vi "Udp Tester ffwd.vi"() -> ()   [LabVIEW 2014]
uses:
  <vilib>/addons/control/pid/pid.llb/PID Lead-Lag (DBL).vi
  <vilib>/addons/control/pid/pid.llb/PID (DBL).vi
  <vilib>/addons/control/pid/pid.llb/PID Percentage to EGU (DBL).vi
  <vilib>/FPGAPlugInAG/myRIO-1900/niLvFpga_Open_myRIO-1900.vi
  <vilib>/rvi/interface/common/dynamic/niFpgaDynamicAddResources.vi
  <vilib>/Utility/error.llb/Error Cluster From Error Code.vi
  <vilib>/rvi/errors/niLvFpgaAdjustHostInterfaceError.vi
  <vilib>/FPGAPlugInAG/Dynamic/niLvFpga_Close_Dynamic.vi
  <vilib>/rvi/interface/nirviOpenFPGA/nirviOpenFPGA.xnode
  FPGA Bitfiles/Test_FPGATarget_CurrentControl_60eBuCSPTsI.lvbitx
  Current Control.vi
  <vilib>/rvi/interface/nirviReadWriteControl/nirviReadWriteControl.xnode
  <vilib>/rvi/interface/nirviCloseFPGA/nirviCloseFPGA.xnode
  <vilib>/rvi/interface/Simulation/niFpgaSimulationCallBeginRW.vi
  <vilib>/Utility/file.llb/Write To Spreadsheet File (I64).vi
  <vilib>/addons/control/pid/NI_PID_pid.lvlib
  <vilib>/ptbypt/NI_PtbyPt.lvlib
  NiFpgaLv.dll
panel:
  in  "output range":cluster{"output high":dbl, "output low":dbl}={"output high"=100.0, "output low"=-100.0} {"output low" format="%.2f"; "output high" format="%.2f"}
  out "SP1:":dbl(slide)=40.87020302841148 min=0.0 max=0.0 scale=0.0..100.0
  in  "Feedforward\nLag Time (min)":dbl(slide)=0.9102981779915218 scale=0.01..10.0
  out "SP and PV":cluster{"Plant Output":dbl, "SP:":dbl}(graph)
  out "MV (mA)":dbl(graph)=20.39115328927357
  in  "Loop Cycle":i32
  in  "Tab Control":enum32{"Profile", "Diagram"}(tab)
  out "Inflow Profile Graph":cluster{dbl, dbl}[](graph)
  in  "Apply Inflow Profile":bool=TRUE
  in  "Constant Flow (%)":dbl=40.0
  in  "Inflow Profile":cluster{"time (s)":dbl, "setpoint":dbl}[](array[cluster])=[{"time (s)"=0.0, "setpoint"=40.0}, {"time (s)"=10.0, "setpoint"=40.0}, {"time (s)"=10.0, "setpoint"=60.0}, {"time (s)"=20.0, "setpoint"=60.0}]
  out "FT Valve":dbl(knob)=84.28886007445381 scale=0.0..190.0
  out "control valve":dbl=86.66603993277398 format="%.2f"
  out "Valve":bool
  out "Pump":bool=TRUE
  out "Bladder Tank":dbl(slide)=49.279730305904245 scale=0.0..100.0 scale format="%.2f"
  out "FT":dbl(knob)=84.28886007445381 scale=0.0..100.0
  out "PV 1":dbl=49.279730305904245
  in  "Stop":bool
  in  "PID parameters (LC)":T1={"Kc"=-20.0, "Ti (min)"=0.1, "Td (min)"=0.0} {"Td (min)" format="%#.6f"; "Ti (min)" format="%#.4f"; "Kc" format="%#.4f"}
  out "PV1:":dbl(slide)=50.762476114859936 scale=0.0..190.0
  out "MV1:":dbl(slide)=100.0 scale=-100.0..100.0
  out "Status?":bool
  # "Time (s)"
  # "Flow (%)"
  # "SP"
  # "///"
  # "///"
  # "///"
  # "1"
  # "///"
  # "SP"
  # "2"
  # "mA"
  # "mA"
  # "FC"
  # "LT"
  # "1"
  # "+"
  # "+"
  # "S"
  # "LC"
  # "FT"
  # "1"
  # "%"
  # "%"
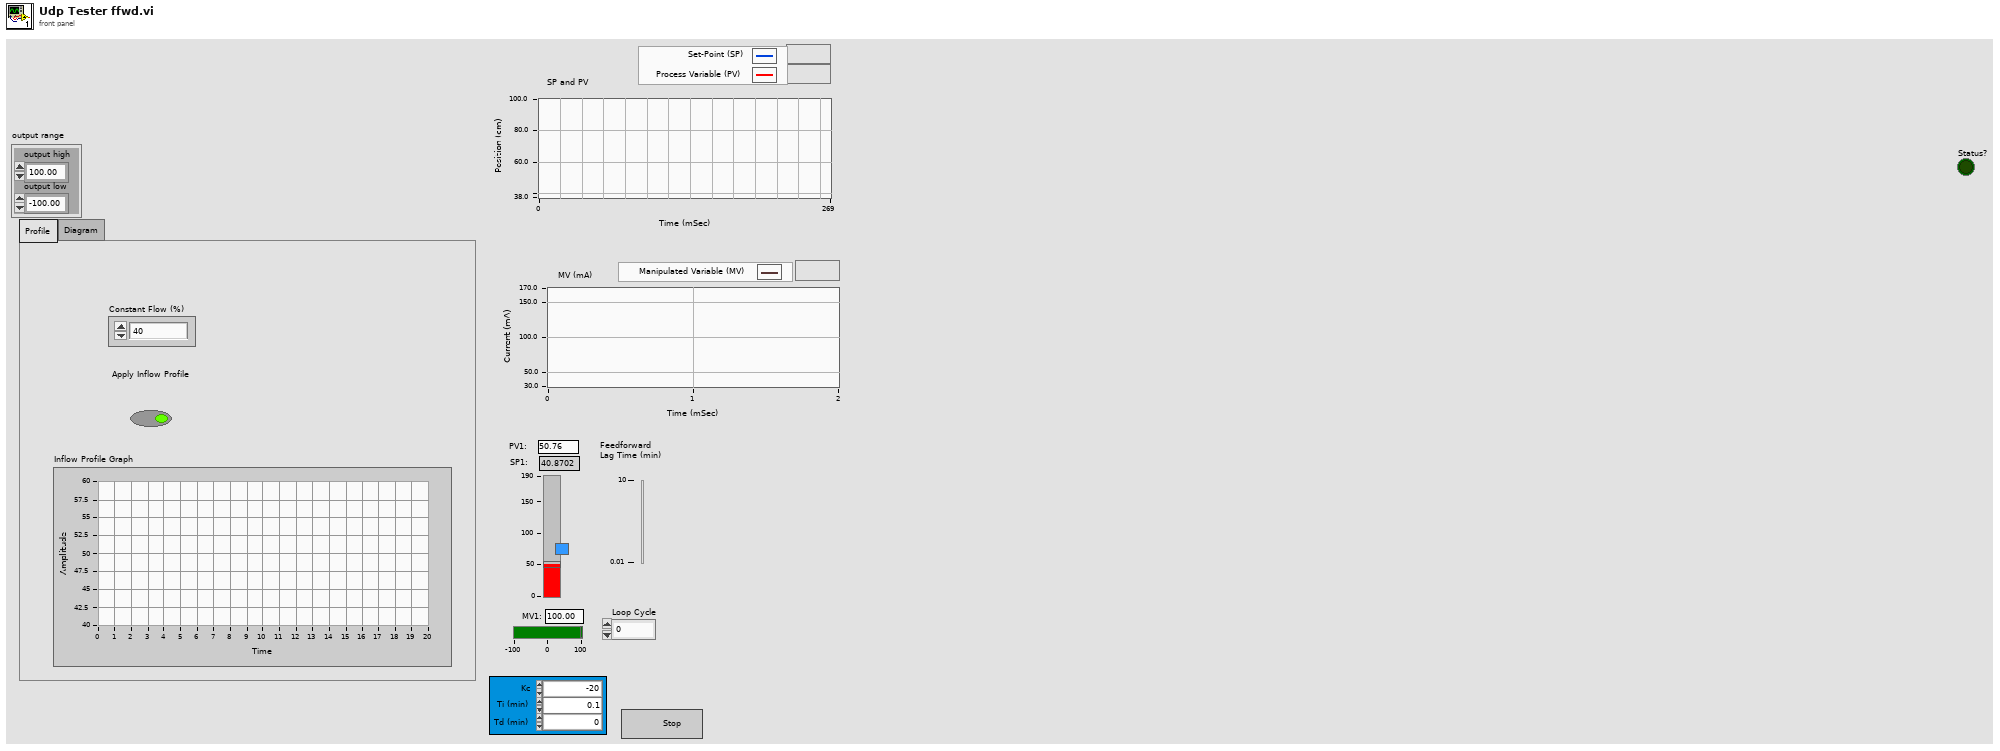
[diagram p1: front panel]
types:
  T1 = cluster{"Kc":dbl, "Ti (min)":dbl, "Td (min)":dbl}
  T2 = enum16{"big-endian, network order", "native, host order", "little-endian"}
  T3 = cluster{"gain":dbl, "lag time (min)":dbl, "lead time (min)":dbl}
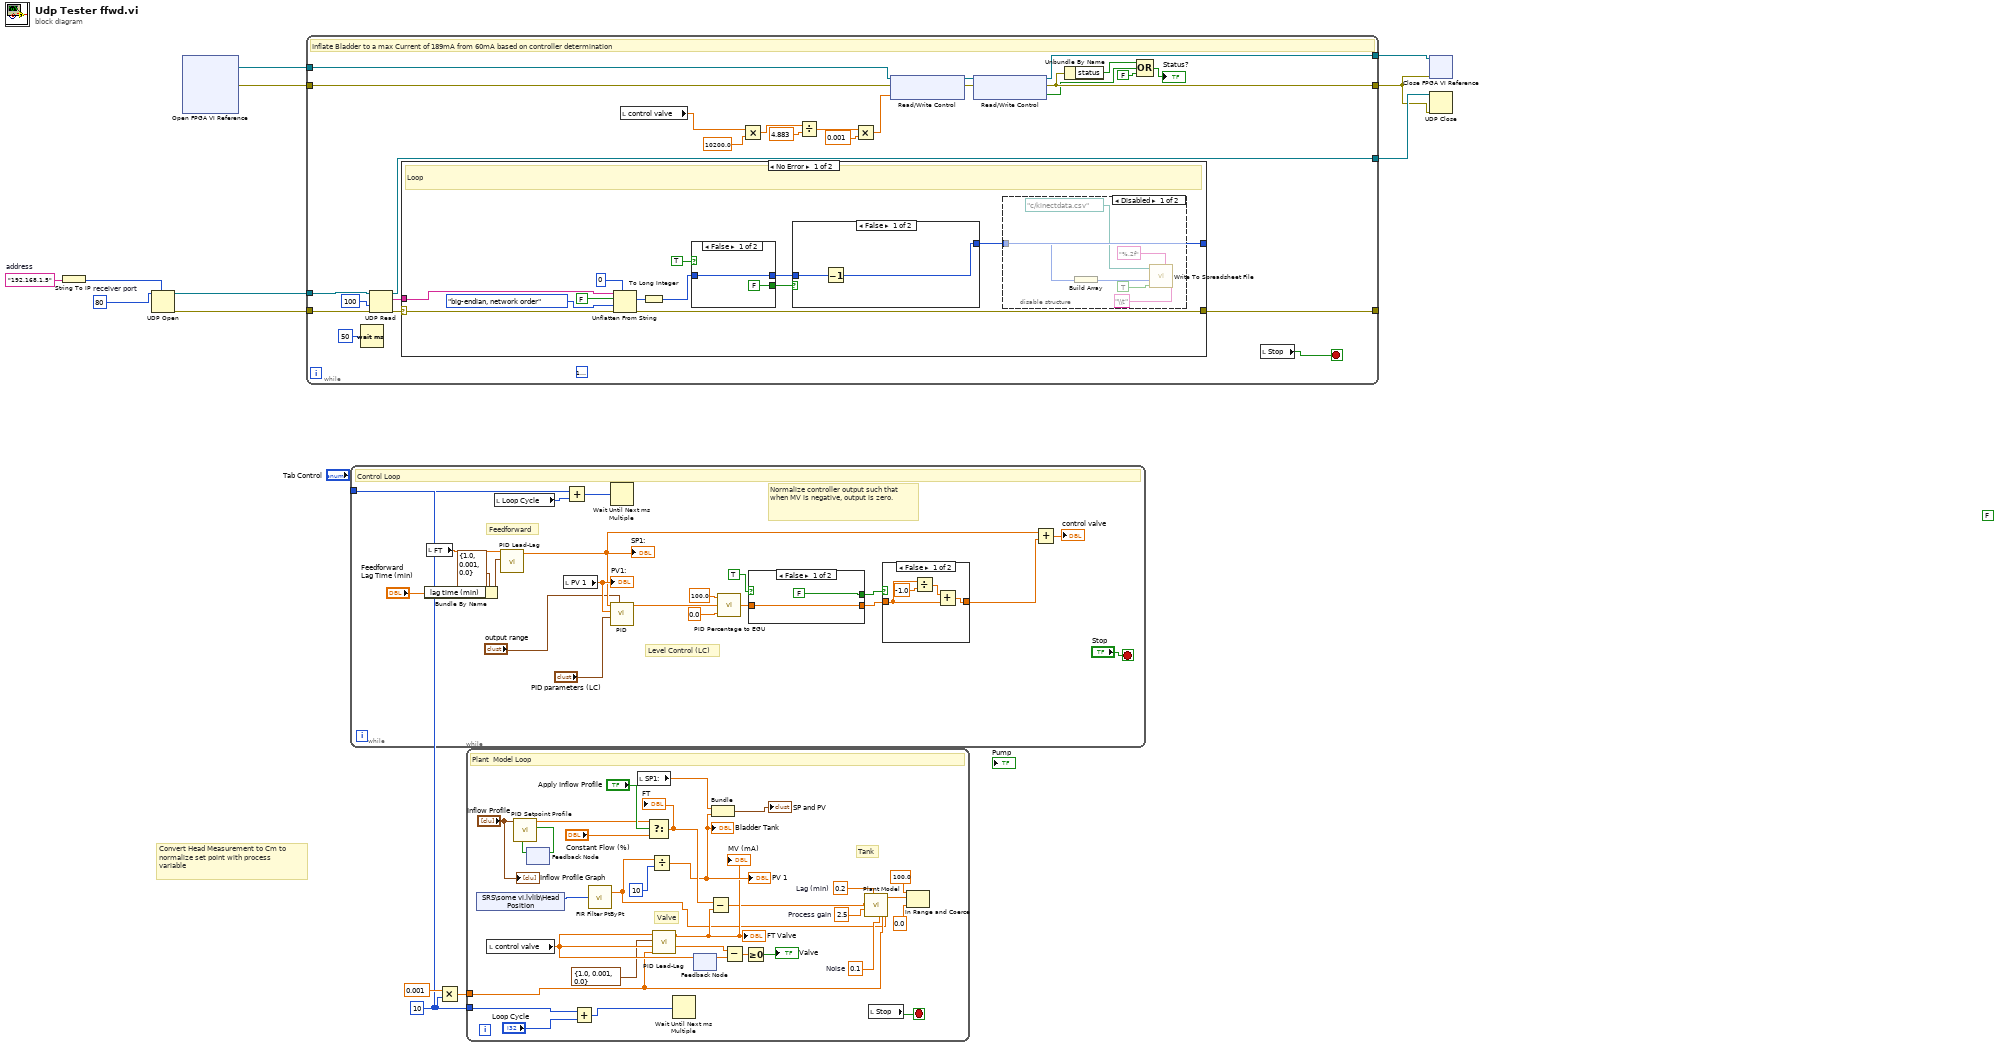
[diagram p0: block diagram]
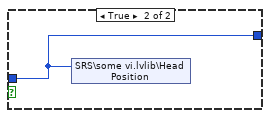
[diagram p3: hidden frame]
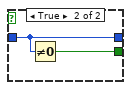
[diagram p4: hidden frame]
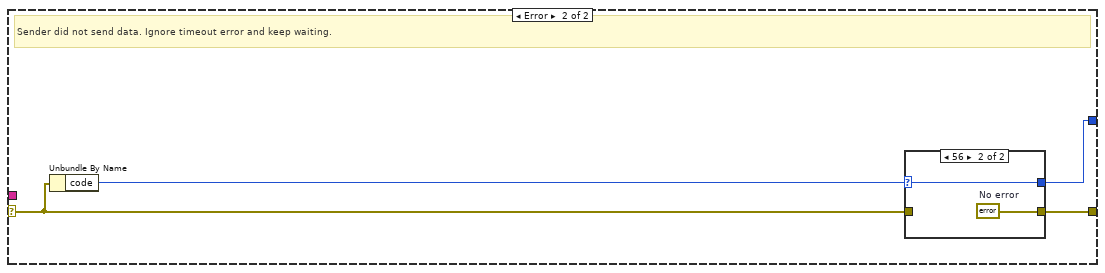
[diagram p5: hidden frame]
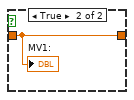
[diagram p7: hidden frame]
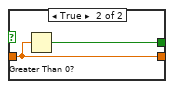
[diagram p8: hidden frame]
diagram:
  w1 = 10
  (unwired) FALSE
  w12 = "192.168.1.5"  # address
  w11 = u16 80  # receiver port
  # "Convert Head Measurement to Cm to normalize set point with process variable"
  n1 = String To IP(1:w12) -> (0:w13:u32)
  n2 = UDP Open(7:w13, 11:w11) -> (port=w10:refnum<k16>, 0:w9:errorcluster)  [unwired: 3 in, 1 out]
  n3 = xnode "Open FPGA VI Reference"() -> ("FPGA VI Reference Out"=w5:refnum<k20>, "error out"=w4:errorcluster)  [unwired: 2 in]
  n4 = while {
    tunnel: w10 -> [w39]
    tunnel: w9 -> [w38]
    tunnel: w5 -> [w33]
    tunnel: [w34] -> w7
    tunnel: w4 -> [w36]
    tunnel: [w35] -> w6
    tunnel: [w18] -> _
    tunnel: [w17] -> w8
    stop <- w14 stop-if-true
    (unwired) u32 16777216
    # "Inflate Bladder to a max Current of 189mA from 60mA based on controller determination"
    n5 = Wait (ms)(milliseconds to wait=u32 50) -> ()  [unwired: 1 out]
    n6 = UDP Read(connection ID=w39, timeout ms (25000)=100, 8:w38) -> (data out=w20:string, error out=w19:errorcluster, 3:w17:refnum<k16>)  [unwired: 3 out]
    n7 = case shown="No Error" w19 {
      selector: w19 -> [w46 w67]
      tunnel: w20 -> [w47 _]
      tunnel: [w45 w66] -> w18
      tunnel: [w41 w65] -> _
      frame No Error {
        # "Loop"
        n8 = Unflatten From String(type=0, binary string=w47, data includes array or string size? (T)=FALSE, byte order (0:big-endian, network order)=T2."big-endian, network order" ("byte order"), error in (no error)=w46) -> (value=w48:i32, error out=w45:errorcluster)  [unwired: 1 out]
        n9 = To Long Integer(number=w48) -> (32bit integer=w43:i32)
        n10 = case shown="False" TRUE {
          tunnel: w43 -> [w61 w63]
          tunnel: [FALSE w64] -> w42
          tunnel: [w61 w63] -> w40
          frame False {
          }
          frame True {
            n11 = Not Equal To 0?(x=w63) -> (x != 0?=w64:bool)
          }
        }
        n12 = case shown="False" w42 {
          tunnel: w40 -> [w59 w60]
          tunnel: [w58 w60] -> w41
          frame False {
            n13 = Decrement(x=w59) -> (x-1=w58:i32)
          }
          frame True {
            n14 = shared-variable "SRS\\some vi.lvlib\\Head Position"(w60) -> ()  [unwired: 1 in, 1 out]
          }
        }
        n15 = disable-structure shown="Disabled" {
          disable-tunnel: w41 -> [w52 _]
          frame Disabled {
            n16 = Build Array(w52) -> (w57:i32[])
            n17 = call-poly <vilib>:"Write To Spreadsheet File.vi"("delimiter (\\t)"="\\t" ("delimiter (\\t)"), "format (%d)"="%.2f", "append to file? (new file:F)"=TRUE, "1D data"=w57, "file path (dialog if empty)"=path "c:/kinectdata.csv") -> ()  [unwired: 3 in, 1 out]
          }
          frame Enabled {
          }
        }
      }
      frame Error {
        # "Sender did not send data. Ignore timeout error and keep waiting."
        n18 = Unbundle By Name(w67) -> ("code"=w68:i32)
        n19 = case shown="56" w68 {
          selector: w68 -> [w69 w71]
          tunnel: w67 -> [w70 _]
          tunnel: [w70 w72] -> w66
          tunnel: [w69 w71] -> w65
          frame Default {
          }
          frame 56 {
            w72 = errorcluster {"status"=FALSE, "code"=0, "source"=""}  # No error
          }
        }
      }
    }
    n20 = local read "control valve"() -> (w15:dbl)
    n21 = Multiply(x=w15, y=10200.0) -> (x*y=w21:dbl)
    n22 = Divide(x=w21, y=4.883) -> (x/y=w24:dbl)
    n23 = Multiply(x=w24, y=0.001) -> (x*y=w30:dbl)
    n24 = xnode "Read/Write Control"("FPGA VI Reference In"=w33, "error in"=w36, "DAC Inlet Valve"=w30) -> ("FPGA VI Reference Out"=w32:refnum<k20>, "error out"=w31:errorcluster)
    n25 = xnode "Read/Write Control"("FPGA VI Reference In"=w32, "error in"=w31) -> ("FPGA VI Reference Out"=w34:refnum<k20>, "error out"=w35:errorcluster, "Inlet Overflow?"=w29:bool)
    n26 = Unbundle By Name(w35) -> ("status"=w27:bool)
    n27 = Compound Arithmetic op=OR(w27, w29, FALSE ("value")) -> (→"Status?":bool)
    n28 = local read "Stop"() -> (w14:bool)
  }
  n29 = while {
    tunnel: w1 -> [w89]
    stop <- "Stop" stop-if-true
    # "Feedforward"
    # "Normalize controller output such that when MV is negative, output is zero."
    # "Level Control (LC)"
    # "Control Loop"
    n30 = Bundle By Name(cluster=T3 {"gain"=1.0, "lag time (min)"=0.001, "lead time (min)"=0.0} ("tuning parameters"), "lag time (min)"="Feedforward\nLag Time (min)") -> (w78:T3)
    n31 = local read "FT"() -> (w75:dbl)
    n32 = local read "Loop Cycle"() -> (w88:i32)
    n33 = call-poly <vilib>:"PID Lead-Lag.vi"("tuning parameters"=w78, "input"=w75) -> ("output"=w74:dbl)  [unwired: 6 in, 1 out]
    "SP1:" <- w74
    n34 = local read "PV 1"() -> (w91:dbl)
    "PV1:" <- w91
    n35 = Add(x=w89, y=w88) -> (x+y=w87:i32)
    n36 = Wait Until Next ms Multiple(millisecond multiple=w87) -> ()  [unwired: 1 out]
    n37 = call-poly <vilib>:"PID.vi"("output range"="output range", "PID gains"="PID parameters (LC)", "process variable"=w91, "setpoint"=w74) -> ("output"=w82:dbl)  [unwired: 6 in, 1 out]
    n38 = call-poly <vilib>:"PID Percentage to EGU.vi"("minimum (EGU)"=0.0, "% span"=w82, "maximum (EGU)"=100.0) -> ("output (EGU)"=w81:dbl)  [unwired: 1 in]
    n39 = case shown="False" TRUE {
      tunnel: w81 -> [w100 w102]
      tunnel: [FALSE w101] -> w85
      tunnel: [w100 w102] -> w84
      frame False {
      }
      frame True {
        n40 = Greater Than 0?(x=w102) -> (x > 0?=w101:bool)
      }
    }
    n41 = case shown="False" w85 {
      tunnel: w84 -> [w95 w98]
      tunnel: [w94 w98] -> w83
      frame False {
        n42 = Divide(x=w95, y=-1.0) -> (x/y=w97:dbl)
        n43 = Add(x=w97, y=w95) -> (x+y=w94:dbl)
      }
      frame True {
        "MV1:" <- w98
      }
    }
    n44 = Add(x=w74, y=w83) -> (x+y=→"control valve":dbl)
  }
  n45 = Multiply(x=0.001, y=w1) -> (x*y=w2:dbl)
  n46 = while {
    tunnel: w2 -> [w107]
    tunnel: w1 -> [w117]
    stop <- w131 stop-if-true
    w109 = 0.2  # Lag (min)
    w105 = 2.5  # Process gain
    w104 = 0.1  # Noise
    # "Tank"
    # "Valve"
    # "Plant  Model Loop"
    n47 = shared-variable "SRS\\some vi.lvlib\\Head Position"() -> (w110:i32)  [unwired: 1 in, 1 out]
    n48 = local read "control valve"() -> (w113:dbl)
    n49 = feedback #1() -> (w132:bool)  [unwired: 1 in]
    n50 = call <vilib>:"PID Setpoint Profile.vi"("reinitialize? (F)"=w132, "setpoint profile"="Inflow Profile") -> ("profile complete?"=w133:bool, "setpoint"=w126:dbl)  [unwired: 4 in, 2 out]
    n51 = feedback-in #1(w133) -> ()
    n52 = Add(x=w117, y="Loop Cycle") -> (x+y=w118:i32)
    n53 = call <vilib>:"FIR Filter PtByPt.vi"("x"=w110) -> ("Filtered x"=w103:dbl)  [unwired: 3 in, 1 out]
    n54 = local read "SP1:"() -> (w115:dbl)
    n55 = Select(t=w126, s="Apply Inflow Profile", f="Constant Flow (%)") -> (s? t:f=w127:dbl)
    "FT" <- w127
    n56 = Divide(x=w103, y=10 ("x")) -> (x/y=w120:dbl)
    "Bladder Tank" <- w120
    "PV 1" <- w120
    n57 = call-poly <vilib>:"PID Lead-Lag.vi"("dt (s)"=w107, "tuning parameters"=T3 {"gain"=1.0, "lag time (min)"=0.001, "lead time (min)"=0.0}, "input"=w113) -> ("output"=w112:dbl)  [unwired: 5 in, 1 out]
    "FT Valve" <- w112
    "MV (mA)" <- w112
    n58 = Wait Until Next ms Multiple(millisecond multiple=w118) -> ()  [unwired: 1 out]
    n59 = feedback-in #2(w113) -> ()
    n60 = feedback #2() -> (w123:dbl)  [unwired: 1 in]
    n61 = Subtract(x=w127, y=w112) -> (x-y=w106:dbl)
    n62 = Bundle("SP1:"=w115, w120) -> (→"SP and PV":cluster{"SP1:":dbl, dbl})  [unwired: 1 in]
    n63 = Subtract(x=w113, y=w123) -> (x-y=w122:dbl)
    n64 = Greater Or Equal To 0?(x=w122) -> (x >= 0?=→"Valve":bool)
    n65 = call "Plant Model.vi"("Initial PV"=w103, "dt (s)"=w107, "Controller Noise (%)"=w104, "Lag (min)"=w109, "Process Gain"=w105, "Manipulated Variable (Output, %)"=w106) -> ("Process Variable (%)"=w108:dbl)  [unwired: 5 in]
    n66 = local read "Stop"() -> (w131:bool)
    n67 = In Range and Coerce(upper limit=100.0, x=w108, lower limit=0.0) -> ()  [unwired: 2 out]
    "Inflow Profile Graph" <- "Inflow Profile"
  }
  n68 = xnode "Close FPGA VI Reference"("FPGA VI Reference In"=w7, "error in"=w6) -> ()  [unwired: 1 out]
  n69 = UDP Close(connection ID=w8, 8:w6) -> ()  [unwired: 2 out]
